vi "Convert ASCII to Measurement Data.vi"(8 "error in (no error)":errorcluster, 10 "Measurement ASCII Data (\"\")":string, 11 "VISA resource name":refnum<visa-resource-name>) -> (0 "error out":errorcluster, 1 "Data":dbl[](array[numeric]) format="%.4f", 2 "Channel":string[](array[string]), 3 "VISA resource name out":refnum<visa-resource-name>, 4 "Unit":string[](array[string]), 5 "Data Status":i32[](array[ring]) items=["Normal", "Differential Input", "Skip", "Over", "Error", "Burnout"], 6 "Alarm Status":i32[][](array[ring]) items=["No Alarm", "High Limit Alarm (H)", "Low Limit Alarm (L)", "Difference High Limit Alarm (h)", "Difference Low Limit Alarm (l)", "High Limit on Rate-of-change Alarm (R)", "Low Limit on Rate-of-change Alarm (r)", "Delay High Limit Alarm (T)", "Delay Low Limit Alarm (t)"], 7 "Date Time":timestamp=timestamp(3345116400 s since 1904-01-01) format="%<%H:%M:%S%3u\n%x>T")   [LabVIEW 2020, in "Yokogawa GX Series.lvlib"]
doc: "This VI converts Measurement ASCII Data to array of data parts."
uses:
  <instrlib>/Yokogawa GX Series/Yokogawa GX Series.lvlib
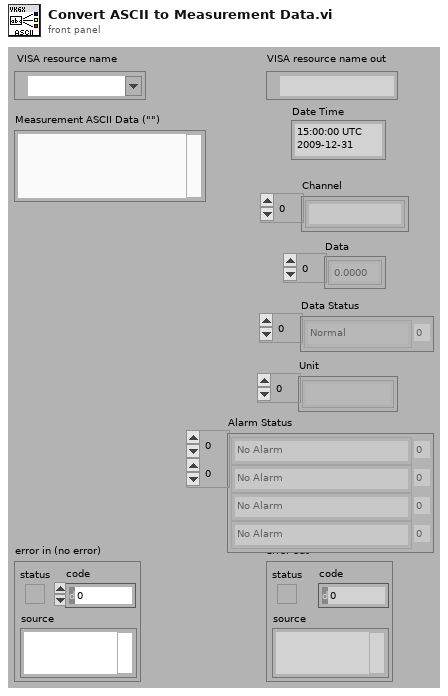
[diagram p1: front panel]
types:
  T1 = typedef "LVDateTimeRec.ctl" = cluster{"fractional second":dbl, "second":i32, "minute":i32, "hour":i32, "day of month":i32, "month":i32, "year":i32, "day of week":i32, "day of year":i32, "DST":i32}
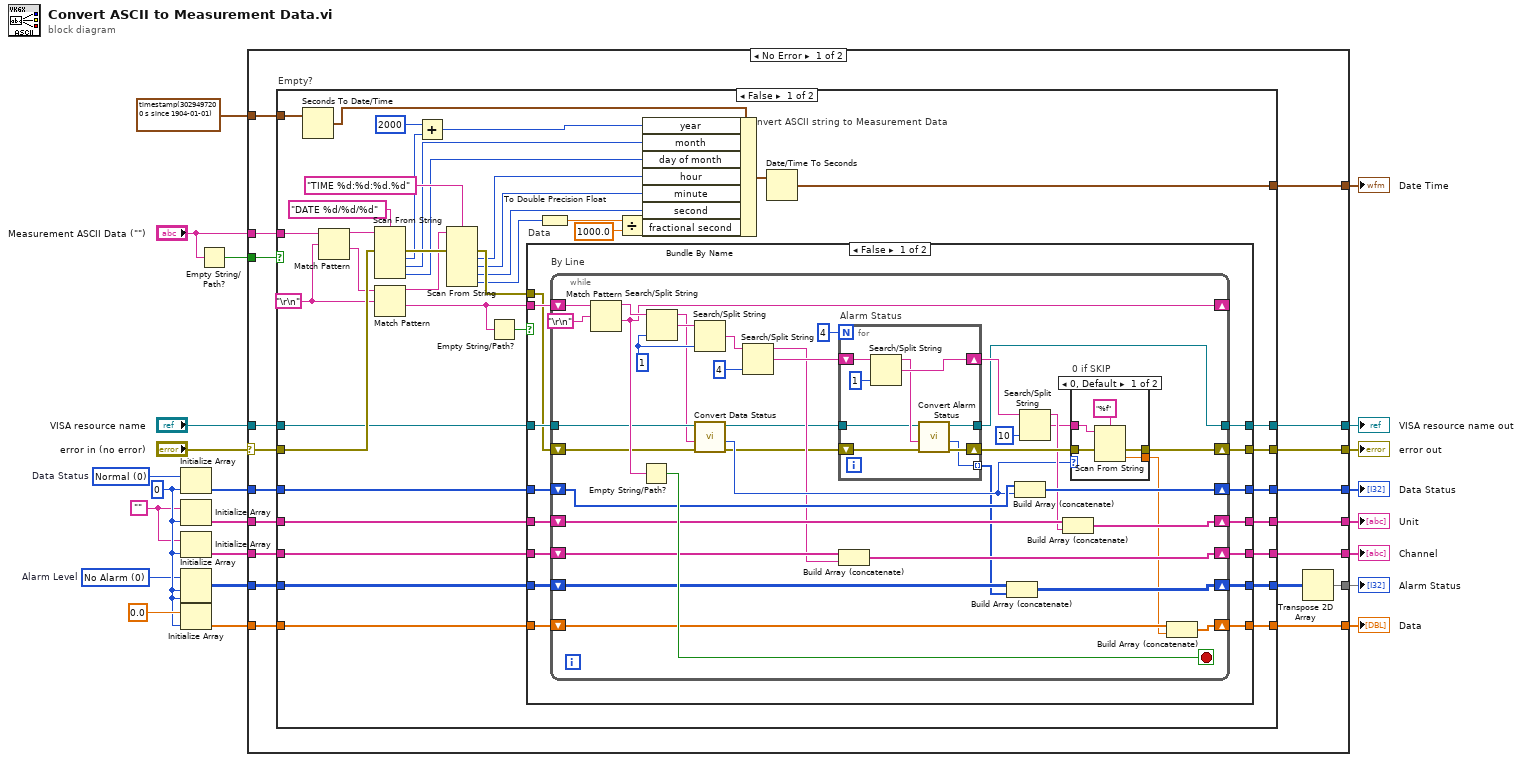
[diagram p0: block diagram]
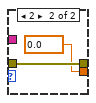
[diagram p2: hidden frame]
diagram:
  w3 = 0 items=["No Alarm", "High Limit Alarm (H)", "Low Limit Alarm (L)", "Difference High Limit Alarm (h)", "Difference Low Limit Alarm (l)", "High Limit on Rate-of-change Alarm (R)", "Low Limit on Rate-of-change Alarm (r)", "Delay High Limit Alarm (T)", "Delay Low Limit Alarm (t)"]  # Alarm Level
  w4 = 0 items=["Normal", "Differential Input", "Skip", "Over", "Error", "Burnout"]  # Data Status
  w2 = ""
  w5 = 0
  n1 = Initialize Array(w4, w5) -> (w20:i32[])
  n2 = Initialize Array(w2, w5) -> (w16:string[])
  n3 = Initialize Array(w2, w5) -> (w19:string[])
  n4 = Initialize Array(w3, w5, w5) -> (w18:i32[][])
  n5 = Initialize Array(0.0, w5) -> (w15:dbl[])
  n6 = Empty String/Path?(string/path="Measurement ASCII Data (\"\")") -> (empty?=w23:bool)
  n7 = case shown="No Error" "error in (no error)" {
    selector: "error in (no error)" -> [w24 w172]
    tunnel: w23 -> [w42 _]
    tunnel: "Measurement ASCII Data (\"\")" -> [w41 _]
    tunnel: "VISA resource name" -> [w40 w173]
    tunnel: w20 -> [w39 w171]
    tunnel: w19 -> [w38 w169]
    tunnel: w18 -> [w37 w168]
    tunnel: w16 -> [w36 w170]
    tunnel: w15 -> [w35 w167]
    tunnel: [w34 w173] -> w14
    tunnel: [w33 w172] -> w13
    tunnel: [w32 w167] -> w12
    tunnel: [w30 w170] -> w11
    tunnel: [w29 w171] -> w10
    tunnel: [w28 w169] -> w9
    tunnel: timestamp(3029497200 s since 1904-01-01) ("Timestamp") -> [w27 w174]
    tunnel: [w26 w174] -> w7
    tunnel: [w25 w168] -> w6
    frame No Error {
      n8 = case "Empty?" shown="False" w42 {
        tunnel: w24 -> [w82 w164]
        tunnel: w39 -> [w75 w166]
        tunnel: [w66 w166] -> w29
        tunnel: [w69 w163] -> w28
        tunnel: w37 -> [w64 w162]
        tunnel: [w71 w162] -> w31
        tunnel: w36 -> [w63 w161]
        tunnel: [w70 w161] -> w30
        tunnel: w35 -> [w62 w160]
        tunnel: [w72 w160] -> w32
        tunnel: w41 -> [w76 _]
        tunnel: [w68 w164] -> w33
        tunnel: w40 -> [w74 w165]
        tunnel: [w67 w165] -> w34
        tunnel: w38 -> [w65 w163]
        tunnel: w27 -> [w46 w159]
        tunnel: [w54 w159] -> w26
        frame False {
          w53 = "\r\n"
          # "Convert ASCII string to Measurement Data"
          n9 = Seconds To Date/Time(time stamp (now)=w46) -> (date time rec=w45:T1)  [unwired: 1 in]
          n10 = Match Pattern(string=w76, regular expression=w53) -> (before substring=w83:string, after substring=w80:string)  [unwired: 3 out]
          n11 = Scan From String(format string="DATE %d/%d/%d", input string=w83, error in=w82) -> (error out=w81:errorcluster, output 1=w51:i32, output 2=w59:i32, output 3=w58:i32)  [unwired: 1 in, 5 out]
          n12 = Match Pattern(string=w80, regular expression=w53) -> (before substring=w79:string, after substring=w61:string)  [unwired: 3 out]
          n13 = Add(x=2000, y=w51) -> (x+y=w50:i32)
          n14 = Scan From String(format string="TIME %d:%d:%d.%d", input string=w79, error in=w81) -> (error out=w73:errorcluster, output 1=w57:i32, output 2=w56:i32, output 3=w55:i32, output 4=w48:i32)  [unwired: 1 in, 6 out]
          n15 = Empty String/Path?(string/path=w61) -> (empty?=w60:bool)
          n16 = case "Data" shown="False" w60 {
            tunnel: w75 -> [w98 w158]
            tunnel: w61 -> [w97 _]
            tunnel: w74 -> [w96 w157]
            tunnel: w73 -> [w95 w156]
            tunnel: [w94 w152] -> w72
            tunnel: [w93 w154] -> w71
            tunnel: [w92 w153] -> w70
            tunnel: [w91 w155] -> w69
            tunnel: [w90 w156] -> w68
            tunnel: [w89 w157] -> w67
            tunnel: [w88 w158] -> w66
            tunnel: w65 -> [w87 w155]
            tunnel: w64 -> [w86 w154]
            tunnel: w63 -> [w85 w153]
            tunnel: w62 -> [w84 w152]
            frame False {
              n17 = while "By Line" {
                shift-left: w95 -> [w108]
                shift-right: [w114] -> w90
                shift-left: w84 -> [w124]
                shift-right: [w123] -> w94
                shift-left: w85 -> [w126]
                shift-right: [w125] -> w92
                shift-left: w86 -> [w105]
                shift-right: [w120] -> w93
                shift-left: w87 -> [w122]
                shift-right: [w121] -> w91
                shift-left: w98 -> [w128]
                shift-right: [w127] -> w88
                shift-left: w97 -> [w135]
                shift-right: [w110] -> _
                tunnel: w96 -> [w109]
                tunnel: [w103] -> w89
                stop <- w134 stop-if-true
                w131 = 1
                n18 = Match Pattern(string=w135, regular expression="\r\n") -> (before substring=w133:string, after substring=w110:string)  [unwired: 3 out]
                n19 = Empty String/Path?(string/path=w110) -> (empty?=w134:bool)
                n20 = Search/Split String(string=w133, offset (0)=w131) -> (substring before match=w107:string, match + rest of string=w132:string)  [unwired: 2 out]
                n21 = Search/Split String(string=w132, offset (0)=w131) -> (match + rest of string=w130:string)  [unwired: 3 out]
                n22 = call <instrlib>:"Convert Data Status.vi"("error in (no error)"=w108, "Data Status String (\"\")"=w107, "VISA resource name"=w109) -> ("error out"=w99:errorcluster, "Data Status"=w106:i32, "VISA resource name out"=w100:refnum<visa-resource-name>)  [unwired: 6 out]
                n23 = Search/Split String(string=w130, offset (0)=4) -> (substring before match=w101:string, match + rest of string=w115:string)  [unwired: 2 out]
                n24 = for "Alarm Status" {
                  N: 4 -> [_]
                  shift-right: [w150] -> w119
                  shift-left: w115 -> [w151]
                  shift-right: [w147] -> w116
                  shift-left: w99 -> [w146]
                  tunnel: [w144] -> w104 mode=indexing
                  tunnel: [w148] -> w103
                  tunnel: w100 -> [w143]
                  n25 = Search/Split String(string=w151, offset (0)=1) -> (substring before match=w145:string, match + rest of string=w150:string)  [unwired: 2 out]
                  n26 = call <instrlib>:"Convert Alarm Status.vi"("error in (no error)"=w146, "Alarm Status String (\"\")"=w145, "VISA resource name"=w143) -> ("error out"=w147:errorcluster, "Alarm Level"=w144:i32, "VISA resource name out"=w148:refnum<visa-resource-name>)  [unwired: 6 out]
                }
                n27 = Build Array (concatenate)(w122, w101) -> (w121:string[])
                n28 = Build Array (concatenate)(w105, w104) -> (w120:i32[][])
                n29 = Build Array (concatenate)(w128, w106) -> (w127:i32[])
                n30 = Search/Split String(string=w119, offset (0)=10) -> (substring before match=w113:string, match + rest of string=w111:string)  [unwired: 2 out]
                n31 = Build Array (concatenate)(w126, w113) -> (w125:string[])
                n32 = case "0 if SKIP" shown="0, Default" w106 {
                  tunnel: w116 -> [w139 w142]
                  tunnel: [w138 w142] -> w114
                  tunnel: [w137 0.0] -> w112
                  tunnel: w111 -> [w136 _]
                  frame 0, Default {
                    n33 = Scan From String(format string="%f", input string=w136, error in=w139) -> (error out=w138:errorcluster, output 1=w137:dbl)  [unwired: 1 in, 3 out]
                  }
                  frame 2 {
                  }
                }
                n34 = Build Array (concatenate)(w124, w112) -> (w123:dbl[])
              }
            }
            frame True {
            }
          }
          n35 = To Double Precision Float(number=w48) -> (double precision float=w47:dbl)
          n36 = Divide(x=w47, y=1000.0) -> (x/y=w43:dbl)
          n37 = Bundle By Name(cluster=w45, "year"=w50, "month"=w59, "day of month"=w58, "hour"=w57, "minute"=w56, "second"=w55, "fractional second"=w43) -> (w44:T1)
          n38 = Date/Time To Seconds(2:w44) -> (0:w54:timestamp)  [unwired: 1 in]
        }
        frame True {
          # "Empty"
        }
      }
      n39 = Transpose 2D Array(2D array=w31) -> (transposed array=w25:i32[][])
    }
    frame Error {
    }
  }
  "error out" <- w13
  "VISA resource name out" <- w14
  "Unit" <- w11
  "Data Status" <- w10
  "Channel" <- w9
  "Alarm Status" <- w6
  "Data" <- w12
  "Date Time" <- w7
